vi "Data Logger Main.vi"(0 "Server Data":cluster{"Concat Data":bool, "WebDAV Push":bool}, 1 "In Spec":bool[](array[boolean])=[FALSE, FALSE, FALSE, FALSE, FALSE, FALSE], 2 "Current Step":i32=2, 3 "Step Time Left":dbl=0.21101045608520508, 4 "Pump Data":T4={"Voltages"=[0.015201568603515625, 0.00335693359375, 0.003021240234375, 0.12260055541992188, 0.06085968017578125, 0.052234649658203125], "PumpCurrent"=[0.015201568603515625, 0.00335693359375, 0.003021240234375, 0.12260055541992188, 0.06085968017578125, 0.052234649658203125], "Speed"=[0.0, 0.0, 0.0, 0.0, 0.0, 0.0], "ControllerCurrent"=[0.015201568603515625, 0.00335693359375, 0.003021240234375, 0.12260055541992188, 0.06085968017578125, 0.052234649658203125], "Pressure"=[0.015201568603515625, 0.00335693359375, 0.003021240234375, 0.12260055541992188, 0.06085968017578125, 0.052234649658203125], "Flow"=[0.0, 0.0, 0.0, 0.125, 0.0625, 0.0625], "Elapsed Time (Display)"=[7.1, 7.1, 7.1, 458133.45, 458138.85000000003, 458126.75], "Avg Pressure"=0.0, "Avg Speed"=0.0, "Elapsed Time"=[4074.9003000000002, 4074.9003000000002, 4074.9003000000002, 4074.9003000000002, 4074.9003000000002, 4074.9003000000002]} {"Elapsed Time" format="%<%H:%M:%S>t"; "Elapsed Time (Display)" format="%<%H:%M:%S>t"; "Speed" format="%#_4f"; "ControllerCurrent" format="%#.1g"; "Pressure" format="%#.0f"; "Flow" format="%#.0f"; "PumpCurrent" format="%#.1g"; "Voltages" format="%#.0f"}, 5 "Tank Data":T3 {"PS Actual (V):" format="%.2f"; "Temp1" format="%#_2g"; "Temp2" format="%#_2g"}, 6 "Auxiliary Data":T1={"Diagnostic Reading"=[nan, nan, nan, nan, nan, nan], "Auxiliary Flow"=[nan, nan, nan, nan, nan, nan]}, 7 "Record Time (sec)":dbl, 8 "Data Logger Mode":T9=enum."Main", 9 "Data Log Start":T5={"App Config"={"Location"="", "Profiles Path"=path "", "Current Profile"="", "CA Number"="", "Controller Type:"=enum."Kuhnke", "Stagger Time (ms)"=0, "Tank 1 Fuel"="", "Tank 2 Fuel"="", "Serial Numbers"={"Position 1 SN"="", "Position 2 SN"="", "Poaition 3 SN"="", "Position 4 SN"="", "Position 5 SN"="", "Position 6 SN"=""}, "Pumps Present"={"Pump 1"=FALSE, "Pump 2"=FALSE, "Pump 3"=FALSE, "Pump 4"=FALSE, "Pump 5"=FALSE, "Pump 6"=FALSE}, "VoltCtrlRef"="", "VoltageSelect"=FALSE, "Watlow Present"=FALSE, "Temp 1"=0.0, "Temp 2"=0.0, "V_Run PI?"=FALSE, "Voltage Limits"={"V_Step"=1e-05, "V_CmdMax"=0.0, "V_CmdMin"=0.0}, "Voltage Far PI"={"V_FarSlew"=10.0, "V_FarKp"=0.0, "V_FarKi"=0.0}, "Voltage Mid PI"={"V_MidSlew"=10.0, "V_MidKp"=0.0, "V_MidKi"=0.0}, "Voltage Close PI"={"V_CloseSlew"=10.0, "V_CloseKp"=0.0, "V_CloseKi"=0.0}, "Voltage Scale"={"V_FFm"=10.0, "V_FFb"=0.0}, "Voltage Cutoffs"={"V_MidCutoff"=0.0, "V_CloseCutoff"=0.0}, "Pressure Scale"={"Pres_FFm"=0.0, "Pres_FFb"=0.0}, "Temp Format"=0, "Temp Tolerance"=0.0, "Target Voltage"=0.0, "Target Pressure"=0.0, "Data Log Init"={"Data Path"=path "", "Data Log Rate (S/s)"=0, "AKLH Rate (Hours/S)"=0.0, "Sync Time Offset (min)"=0, "IP Last 3"=0, "WebDAV IP"=""}, "Email Handler IP"="", "ADC Check"=FALSE, "3 Pump Tank"=FALSE, "Freq Flow?"=FALSE, "Profile Temp Control"=FALSE, "Read Controller Diag"=FALSE, "FFT Min Freq."=0, "FFT Max Freq."=0, "Speed by Current"=FALSE, "Watlow is F4T?"=FALSE, "Test Stop Time"=0.0, "Stop Time Enable"=TRUE, "Timers Include Off-Time"=FALSE}, "Profile"=[], "Controller Type"="", "Tank CMDs"={"PS CMD"=0.0, "Press CMD"=0.0, "Temp 1 CMD"=0.0, "Temp 2 CMD"=0.0, "AO2 CMD"=0.0}}, 11 "Data Log Init":T8, 13 "Tank CMDs":T2) -> ()   [LabVIEW 2013]
uses:
  Data Logger Mode.ctl
  Data Log Init.ctl
  Data Log Start.ctl
  Type Defs/App Config.ctl
  Type Defs/Controller Names.ctl
  Controls/Tank CMDs.ctl
  Controls/Pump Data.ctl
  Controls/Tank Data.ctl
  Type Defs/Auxiliary Data.ctl
  <userlib>/_OpenG.lib/array/array.llb/Remove Duplicates from 1D Array (String)__ogtk.vi
  <userlib>/_OpenG.lib/array/array.llb/Filter 1D Array (String)__ogtk.vi
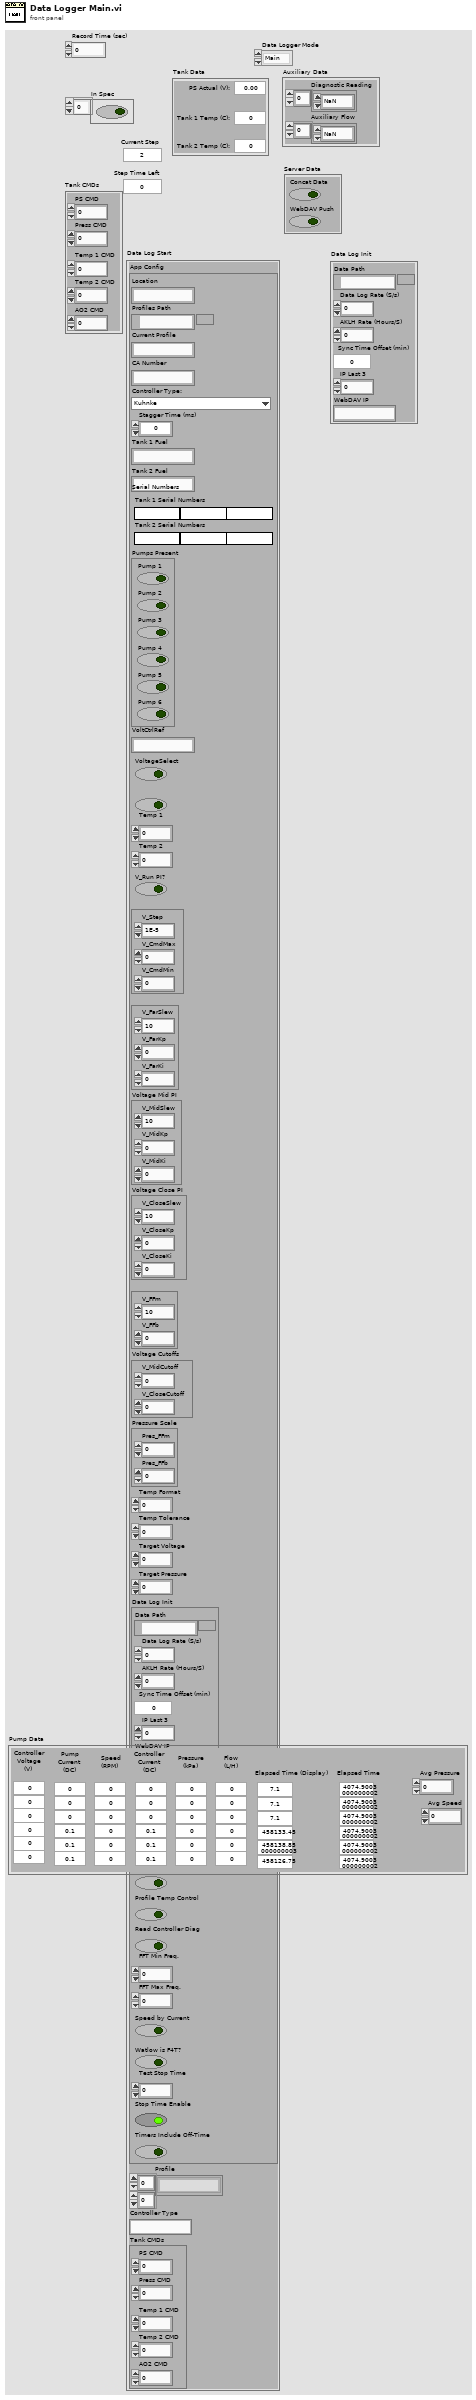
[diagram p1: front panel]
types:
  T1 = typedef "Auxiliary Data.ctl" = cluster{"Diagnostic Reading":dbl[], "Auxiliary Flow":dbl[]}
  T2 = typedef "Tank CMDs.ctl" = cluster{"PS CMD":dbl, "Press CMD":dbl, "Temp 1 CMD":dbl, "Temp 2 CMD":dbl, "AO2 CMD":dbl}
  T3 = typedef "Tank Data.ctl" = cluster{"PS Actual (V):":dbl, "Temp1":dbl, "Temp2":dbl}
  T4 = typedef "Pump Data.ctl" = cluster{"Voltages":dbl[], "PumpCurrent":dbl[], "Speed":dbl[], "ControllerCurrent":dbl[], "Pressure":dbl[], "Flow":dbl[], "Elapsed Time (Display)":dbl[], "Avg Pressure":dbl, "Avg Speed":dbl, "Elapsed Time":dbl[]}
  T5 = typedef "Data Log Start.ctl" = cluster{"App Config":T6, "Profile":string[][], "Controller Type":string, "Tank CMDs":T2}
  T6 = typedef "App Config.ctl" = cluster{"Location":string, "Profiles Path":path, "Current Profile":string, "CA Number":string, "Controller Type:":T7, "Stagger Time (ms)":i32, "Tank 1 Fuel":string, "Tank 2 Fuel":string, "Serial Numbers":cluster{"Position 1 SN":string, "Position 2 SN":string, "Poaition 3 SN":string, "Position 4 SN":string, "Position 5 SN":string, "Position 6 SN":string}, "Pumps Present":cluster{"Pump 1":bool, "Pump 2":bool, "Pump 3":bool, "Pump 4":bool, "Pump 5":bool, "Pump 6":bool}, "VoltCtrlRef":string, "VoltageSelect":bool, "Watlow Present":bool, "Temp 1":dbl, "Temp 2":dbl, "V_Run PI?":bool, "Voltage Limits":cluster{"V_Step":dbl, "V_CmdMax":dbl, "V_CmdMin":dbl}, "Voltage Far PI":cluster{"V_FarSlew":dbl, "V_FarKp":dbl, "V_FarKi":dbl}, "Voltage Mid PI":cluster{"V_MidSlew":dbl, "V_MidKp":dbl, "V_MidKi":dbl}, "Voltage Close PI":cluster{"V_CloseSlew":dbl, "V_CloseKp":dbl, "V_CloseKi":dbl}, "Voltage Scale":cluster{"V_FFm":dbl, "V_FFb":dbl}, "Voltage Cutoffs":cluster{"V_MidCutoff":dbl, "V_CloseCutoff":dbl}, "Pressure Scale":cluster{"Pres_FFm":dbl, "Pres_FFb":dbl}, "Temp Format":i32, "Temp Tolerance":dbl, "Target Voltage":dbl, "Target Pressure":dbl, "Data Log Init":T8, "Email Handler IP":string, "ADC Check":bool, "3 Pump Tank":bool, "Freq Flow?":bool, "Profile Temp Control":bool, "Read Controller Diag":bool, "FFT Min Freq.":i32, "FFT Max Freq.":i32, "Speed by Current":bool, "Watlow is F4T?":bool, "Test Stop Time":dbl, "Stop Time Enable":bool, "Timers Include Off-Time":bool}
  T7 = typedef "Controller Names.ctl" = enum16{"Kuhnke", "Helbako BLDC", "Conti", "Hella BLDC OL PWM", "Hella BLDC Turbine OL PWM", "Hella BLDC Pressure", "Helbako (old)", "TI PWM", "PSA", "Hella Gas", "Hella Diesel", "8 Comm", "10 Comm", "8 Comm Hella", "10 Comm Hella", "8 Comm Omron", "10 Comm Omron", "8 Comm Nissan", "10 Comm Nissan"}
  T8 = typedef "Data Log Init.ctl" = cluster{"Data Path":path, "Data Log Rate (S/s)":u32, "AKLH Rate (Hours/S)":dbl, "Sync Time Offset (min)":i32, "IP Last 3":i32, "WebDAV IP":string}
  T9 = typedef "Data Logger Mode.ctl" = enum16{"Init", "Main", "Start", "Stop"}
  T10 = cluster{"Pump 1":bool, "Pump 2":bool, "Pump 3":bool, "Pump 4":bool, "Pump 5":bool, "Pump 6":bool}
  T11 = cluster{"Data Log Base":path, "AKLH Base":path, "AKLH Today Base":path, "AKLH Sync Base":path, "Data Log Rate (ms)":u32, "AKLH Rate (ms)":u32, "Sync Time (min)":i32, "Profile":string[][], "Target Speeds":string[], "App Config":T6, "AKLH Filenames":string[], "Data Log Dirs":path[], "AKLH Dirs":path[], "AKLH Today Dirs":path[], "AKLH Sync Dirs":path[], "Data Log Hdr Paths":path[], "AKLH Today Hdr Paths":path[], "Log Data":bool, "Data Log Times":u32[], "AKLH Log Times":u32[][], "WebDAV IP":string, "File Check Time (ms)":u32, "File Check Period (ms)":u32, "FC Data Log Times":u32[], "FC AKLH Log Times":u32[][], "Data Log Sizes":i64[], "AKLH Log Sizes":i64[][]}
  T12 = cluster{"Position 1 SN":string, "Position 2 SN":string, "Poaition 3 SN":string, "Position 4 SN":string, "Position 5 SN":string, "Position 6 SN":string}
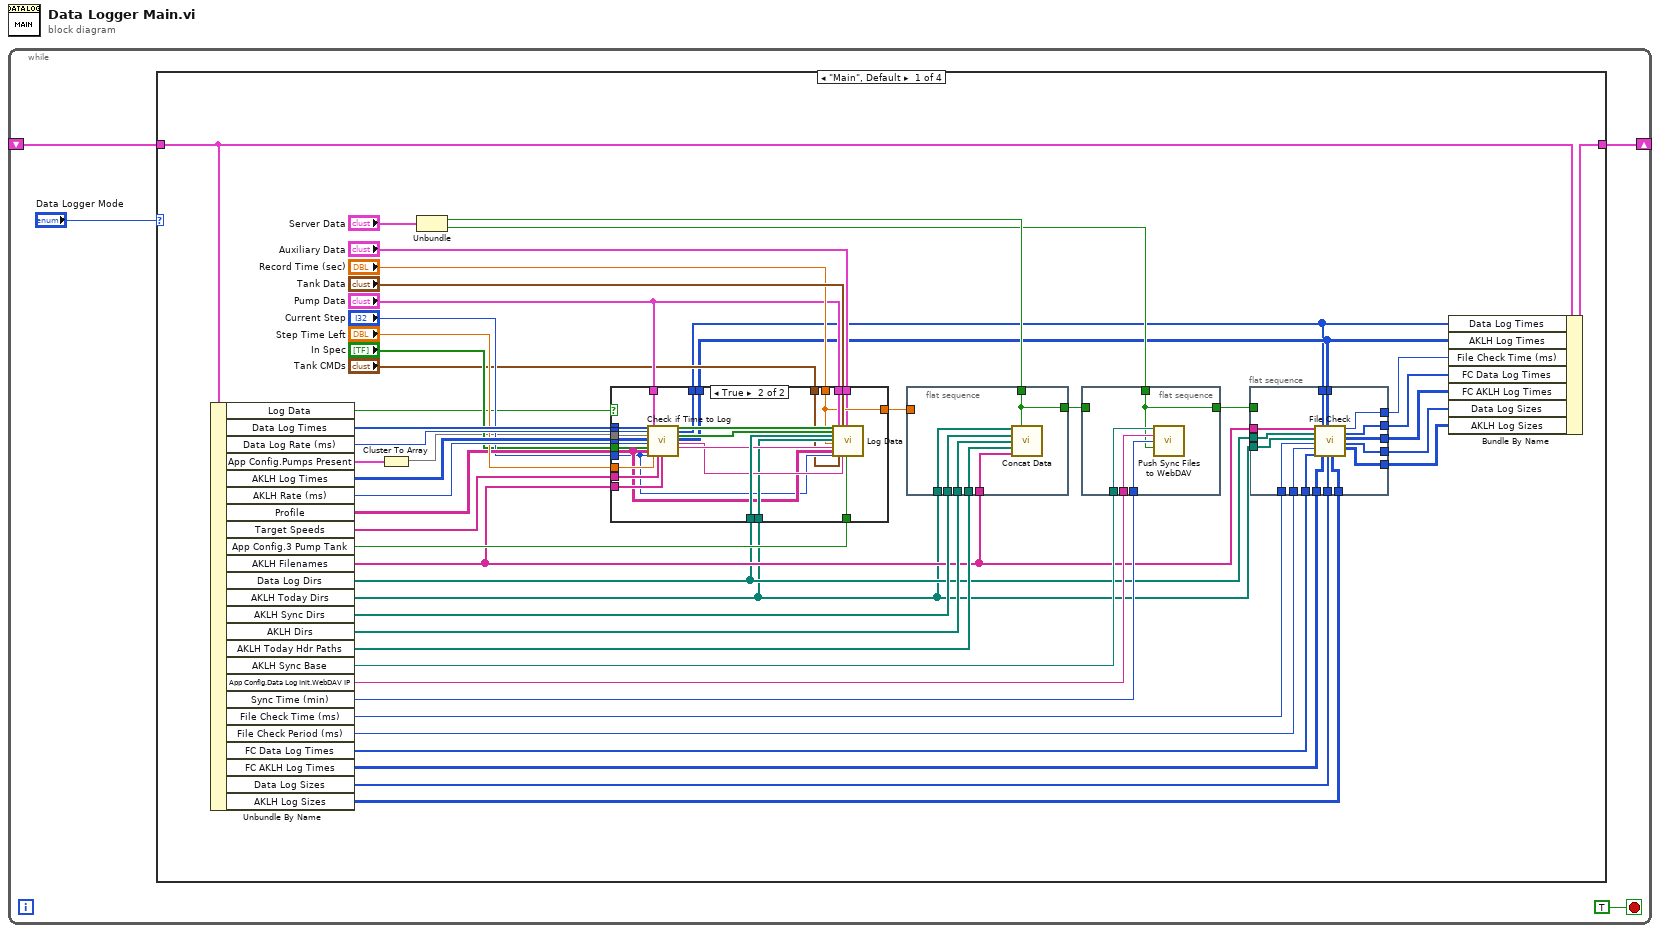
[diagram p0: block diagram]
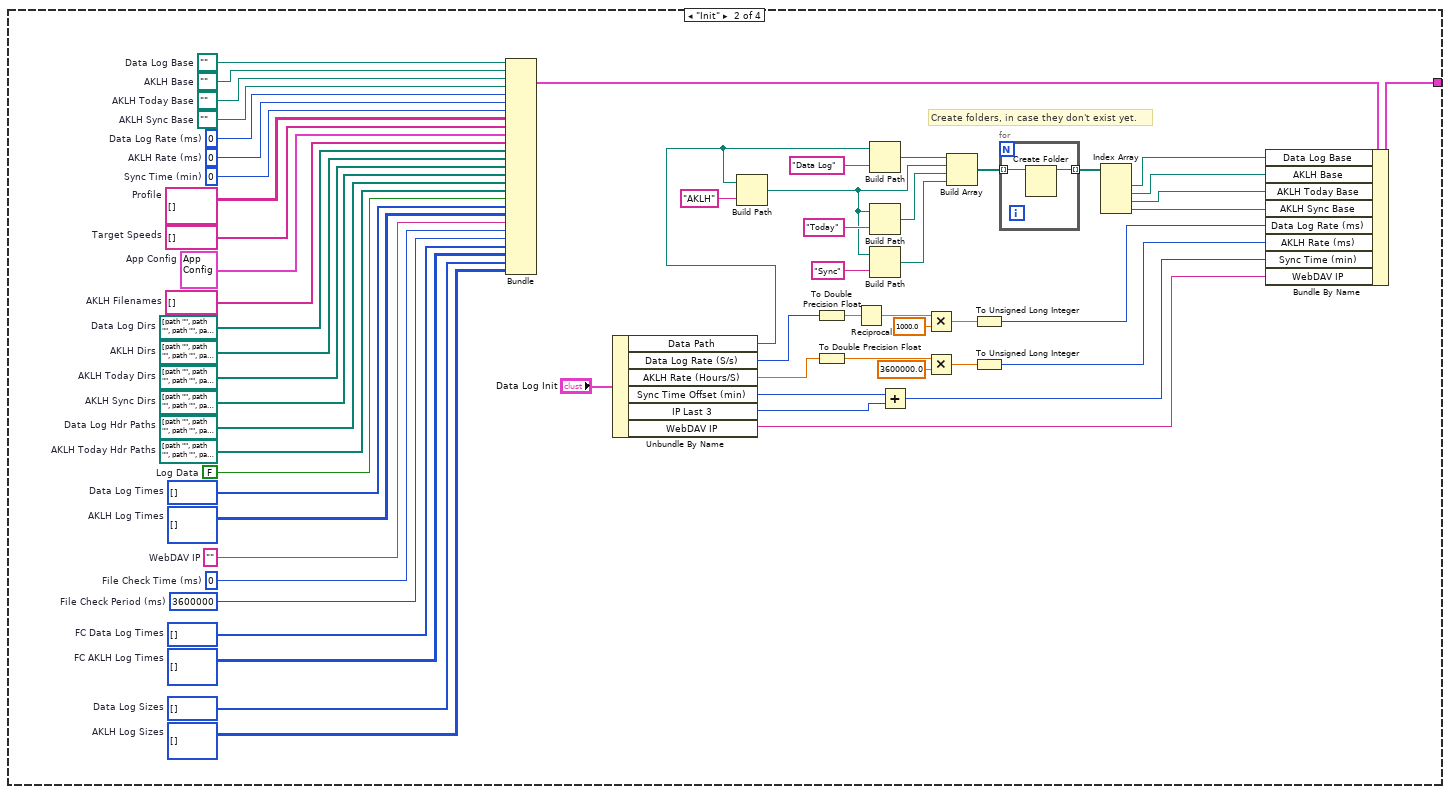
[diagram p3: hidden frame]
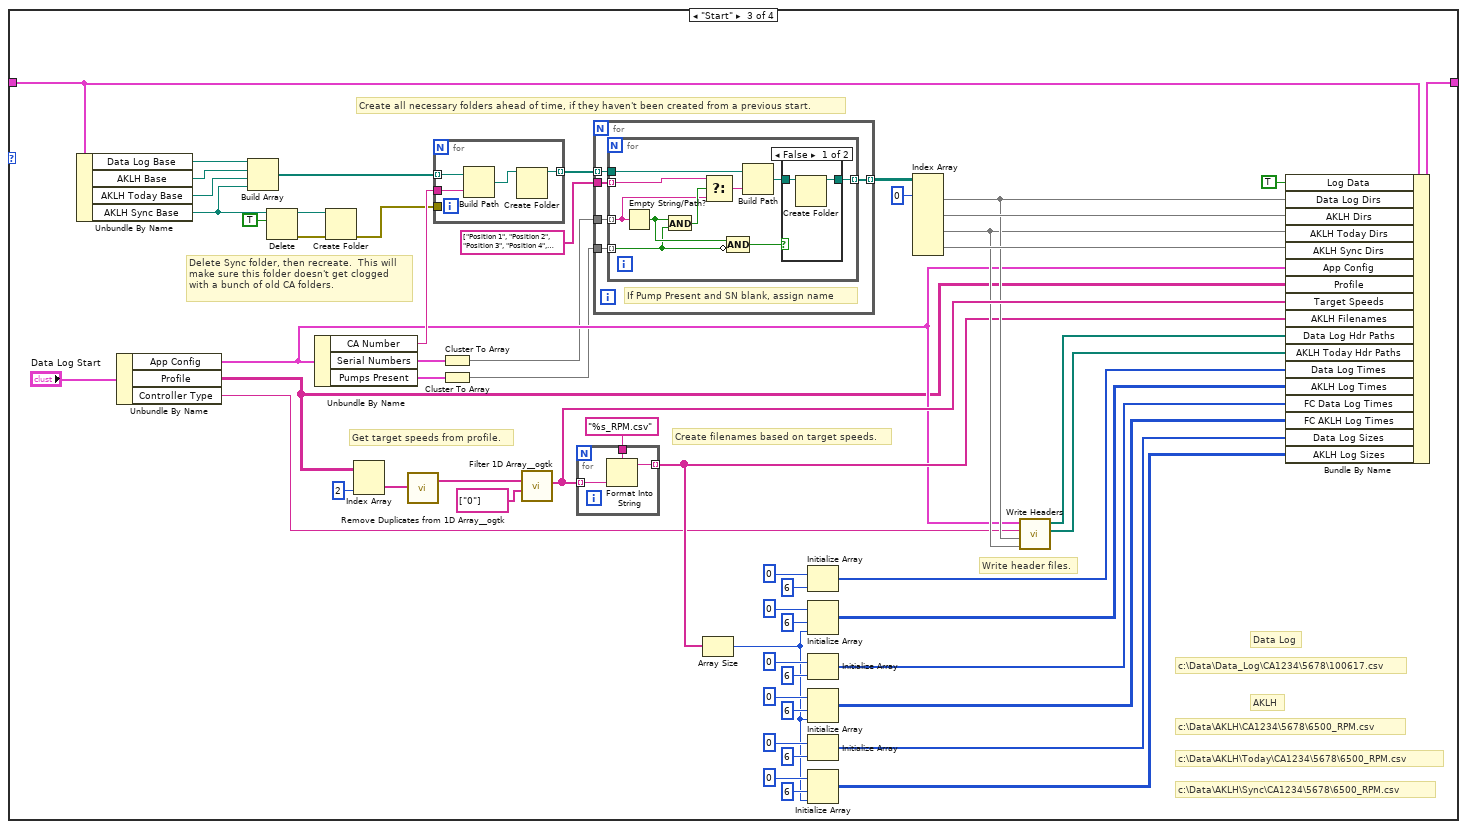
[diagram p4: hidden frame]
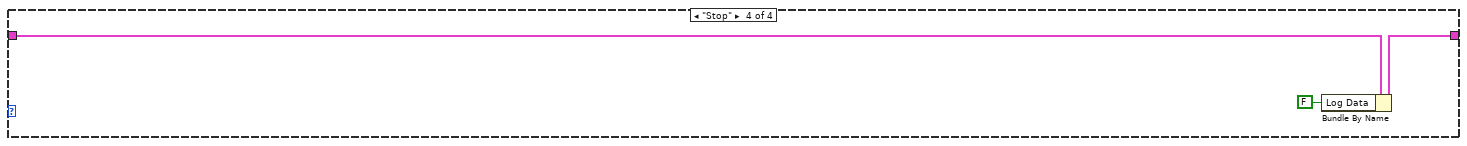
[diagram p6: hidden frame]
diagram:
  n1 = while {
    shift-right: [w2] -> _
    shift-left: _ -> [w1]
    stop <- TRUE stop-if-true
    n2 = case shown="\"Main\", Default" "Data Logger Mode" {
      tunnel: [w51 w160 w212 w253] -> w2
      tunnel: w1 -> [w52 _ w213 w254]
      frame "Main", Default {
        n3 = Unbundle By Name(w52) -> ("Log Data"=w31:bool, "Data Log Times"=w50:u32[], "Data Log Rate (ms)"=w49:u32, "App Config.Pumps Present"=w34:T10, "AKLH Log Times"=w48:u32[][], "AKLH Rate (ms)"=w47:u32, "Profile"=w38:string[][], "Target Speeds"=w45:string[], "App Config.3 Pump Tank"=w28:bool, "AKLH Filenames"=w20:string[], "Data Log Dirs"=w19:path[], "AKLH Today Dirs"=w18:path[], "AKLH Sync Dirs"=w44:path[], "AKLH Dirs"=w43:path[], "AKLH Today Hdr Paths"=w42:path[], "AKLH Sync Base"=w41:path, "App Config.Data Log Init.WebDAV IP"=w40:string, "Sync Time (min)"=w39:i32, "File Check Time (ms)"=w17:u32, "File Check Period (ms)"=w16:u32, "FC Data Log Times"=w15:u32[], "FC AKLH Log Times"=w14:u32[][], "Data Log Sizes"=w13:i64[], "AKLH Log Sizes"=w12:i64[][])
        n4 = Cluster To Array(cluster=w34) -> (array=w33:bool[])
        n5 = Unbundle("Server Data") -> ("Concat Data"=w24:bool, "WebDAV Push"=w23:bool)
        n6 = case shown="True" w31 {
          tunnel: w50 -> [w81 w107]
          tunnel: w49 -> [_ w106]
          tunnel: w48 -> [w80 w105]
          tunnel: w47 -> [_ w104]
          tunnel: "Step Time Left" -> [_ w103]
          tunnel: w45 -> [_ w102]
          tunnel: w19 -> [_ w99]
          tunnel: [w81 w96] -> w10
          tunnel: [w80 w95] -> w11
          tunnel: w18 -> [_ w94]
          tunnel: w20 -> [_ w93]
          tunnel: w38 -> [_ w88]
          tunnel: "Current Step" -> [_ w87]
          tunnel: "Tank Data" -> [_ w92]
          tunnel: "Pump Data" -> [_ w91]
          tunnel: "In Spec" -> [_ w90]
          tunnel: w33 -> [_ w89]
          tunnel: "Record Time (sec)" -> [w79 w86]
          tunnel: [w79 w86] -> w29
          tunnel: w28 -> [_ w85]
          tunnel: "Pump Data" -> [_ w84]
          tunnel: "Tank CMDs" -> [_ w83]
          tunnel: "Auxiliary Data" -> [_ w82]
          frame False {
          }
          frame True {
            n7 = call "Check if Time to Log.vi"("Data Log Times IN"=w107, "Data Log Rate (ms)"=w106, "Pumps Present"=w89, "AKLH Log Times IN"=w105, "AKLH Rate (ms)"=w104, "In Spec"=w90, "Profile"=w88, "Current Step"=w87, "Pump Data"=w84, "Step Time Left"=w103, "Target Speeds"=w102, "AKLH Filenames"=w93) -> ("Log Data"=w101:bool[], "Data Log Times OUT"=w96:u32[], "Log AKLH"=w100:bool[], "AKLH Log Times OUT"=w95:u32[][], "AKLH Filename"=w97:string, "Target Speed"=w98:string)  [unwired: 10 in]
            n8 = call "Log Data.vi"("Log Data"=w101, "Log AKLH"=w100, "Data Log Dirs"=w99, "AKLH Today Dirs"=w94, "Record Time (sec)"=w86, "Target Speed"=w98, "Profile"=w88, "Current Step"=w87, "Pump Data"=w91, "Tank CMDs"=w83, "Tank Data"=w92, "AKLH Filename"=w97, "Auxiliary Data"=w82, "3 Pump Tank"=w85) -> ()  [unwired: 14 in]
          }
        }
        n9 = flat-sequence {
          tunnel: w18 -> [w78]
          tunnel: w44 -> [w77]
          tunnel: w43 -> [w76]
          tunnel: w20 -> [w75]
          tunnel: w42 -> [w74]
          tunnel: w24 -> [w73]
          tunnel: [w73] -> w30
          tunnel: w29 -> [_]
          frame #0 {
            n10 = call "Concat Data.vi"("AKLH Today Dirs"=w78, "Concat Data"=w73, "AKLH Sync Dirs"=w77, "AKLH Dirs"=w76, "AKLH Today Hdr Paths"=w74, "AKLH Filenames"=w75) -> ()  [unwired: 10 in]
          }
        }
        n11 = flat-sequence {
          tunnel: w41 -> [w72]
          tunnel: w40 -> [w71]
          tunnel: w39 -> [w70]
          tunnel: w23 -> [w69]
          tunnel: w30 -> [_]
          tunnel: [w69] -> w21
          frame #0 {
            n12 = call "Push Sync Files to WebDAV.vi"("AKLH Sync Base"=w72, "WebDAV IP"=w71, "Sync Time (min)"=w70, "WebDAV Push"=w69) -> ()  [unwired: 12 in]
          }
        }
        n13 = flat-sequence {
          tunnel: w21 -> [_]
          tunnel: w20 -> [w66]
          tunnel: w19 -> [w65]
          tunnel: w18 -> [w64]
          tunnel: w17 -> [w63]
          tunnel: w16 -> [w62]
          tunnel: w15 -> [w61]
          tunnel: w14 -> [w60]
          tunnel: w13 -> [w58]
          tunnel: w12 -> [w59]
          tunnel: w11 -> [w68]
          tunnel: w10 -> [w67]
          tunnel: [w57] -> w9
          tunnel: [w56] -> w5
          tunnel: [w55] -> w6
          tunnel: [w54] -> w8
          tunnel: [w53] -> w7
          frame #0 {
            n14 = call "File Check.vi"("AKLH Filenames"=w66, "Data Log Dirs"=w65, "AKLH Today Dirs"=w64, "File Check Time (ms) In"=w63, "File Check Period (ms)"=w62, "FC Data Log Times In"=w61, "Data Log Times IN"=w67, "FC AKLH Log Times In"=w60, "AKLH Log Times IN"=w68, "Data Log Sizes In"=w58, "AKLH Log Sizes In"=w59) -> ("File Check Time (ms) Out"=w56:u32, "FC Data Log Times Out"=w55:u32[], "FC AKLH Log Times Out"=w53:u32[][], "Data Log Sizes Out"=w54:i64[], "AKLH Log Sizes Out"=w57:i64[][])  [unwired: 4 in]
          }
        }
        n15 = Bundle By Name(cluster=w52, "Data Log Times"=w10, "AKLH Log Times"=w11, "File Check Time (ms)"=w5, "FC Data Log Times"=w6, "FC AKLH Log Times"=w7, "Data Log Sizes"=w8, "AKLH Log Sizes"=w9) -> (w51:T11)
      }
      frame "Init" {
        w108 = i64[][] []  # AKLH Log Sizes
        w109 = i64[] []  # Data Log Sizes
        w110 = u32[][] []  # FC AKLH Log Times
        w111 = u32[] []  # FC Data Log Times
        w112 = u32 3600000  # File Check Period (ms)
        w113 = u32 0  # File Check Time (ms)
        w130 = ""  # WebDAV IP
        w131 = u32[][] []  # AKLH Log Times
        w132 = u32[] []  # Data Log Times
        w133 = FALSE  # Log Data
        w134 = path[] [path "", path "", path "", path "", path "", path ""]  # AKLH Today Hdr Paths
        w135 = path[] [path "", path "", path "", path "", path "", path ""]  # Data Log Hdr Paths
        w136 = path[] [path "", path "", path "", path "", path "", path ""]  # AKLH Sync Dirs
        w137 = path[] [path "", path "", path "", path "", path "", path ""]  # AKLH Today Dirs
        w138 = path[] [path "", path "", path "", path "", path "", path ""]  # AKLH Dirs
        w139 = path[] [path "", path "", path "", path "", path "", path ""]  # Data Log Dirs
        w140 = string[] []  # AKLH Filenames
        w141 = T6 {"Location"="", "Profiles Path"=path "", "Current Profile"="", "CA Number"="", "Controller Type:"=enum."Kuhnke", "Stagger Time (ms)"=0, "Tank 1 Fuel"="", "Tank 2 Fuel"="", "Serial Numbers"={"Position 1 SN"="", "Position 2 SN"="", "Poaition 3 SN"="", "Position 4 SN"="", "Position 5 SN"="", "Position 6 SN"=""}, "Pumps Present"={"Pump 1"=FALSE, "Pump 2"=FALSE, "Pump 3"=FALSE, "Pump 4"=FALSE, "Pump 5"=FALSE, "Pump 6"=FALSE}, "VoltCtrlRef"="", "VoltageSelect"=FALSE, "Watlow Present"=FALSE, "Temp 1"=0.0, "Temp 2"=0.0, "V_Run PI?"=FALSE, "Voltage Limits"={"V_Step"=0.0, "V_CmdMax"=0.0, "V_CmdMin"=0.0}, "Voltage Far PI"={"V_FarSlew"=0.0, "V_FarKp"=0.0, "V_FarKi"=0.0}, "Voltage Mid PI"={"V_MidSlew"=0.0, "V_MidKp"=0.0, "V_MidKi"=0.0}, "Voltage Close PI"={"V_CloseSlew"=0.0, "V_CloseKp"=0.0, "V_CloseKi"=0.0}, "Voltage Scale"={"V_FFm"=0.0, "V_FFb"=0.0}, "Voltage Cutoffs"={"V_MidCutoff"=0.0, "V_CloseCutoff"=0.0}, "Pressure Scale"={"Pres_FFm"=0.0, "Pres_FFb"=0.0}, "Temp Format"=0, "Temp Tolerance"=0.0, "Target Voltage"=0.0, "Target Pressure"=0.0, "Data Log Init"={"Data Path"=path "", "Data Log Rate (S/s)"=0, "AKLH Rate (Hours/S)"=0.0, "Sync Time Offset (min)"=0, "IP Last 3"=0, "WebDAV IP"=""}, "Email Handler IP"="", "ADC Check"=FALSE, "3 Pump Tank"=FALSE, "Freq Flow?"=FALSE, "Profile Temp Control"=FALSE, "Read Controller Diag"=FALSE, "FFT Min Freq."=0, "FFT Max Freq."=0, "Speed by Current"=FALSE, "Watlow is F4T?"=FALSE, "Test Stop Time"=0.0, "Stop Time Enable"=FALSE, "Timers Include Off-Time"=FALSE}  # App Config
        w143 = string[][] []  # Profile
        w142 = string[] []  # Target Speeds
        w145 = 0  # Sync Time (min)
        w162 = u32 0  # AKLH Rate (ms)
        w163 = u32 0  # Data Log Rate (ms)
        w164 = path ""  # AKLH Sync Base
        w165 = path ""  # AKLH Today Base
        w166 = path ""  # AKLH Base
        w167 = path ""  # Data Log Base
        # "Create folders, in case they don't exist yet."
        n16 = Bundle("Data Log Base"=w167, "AKLH Base"=w166, "AKLH Today Base"=w165, "AKLH Sync Base"=w164, "Data Log Rate (ms)"=w163, "AKLH Rate (ms)"=w162, "Sync Time (min)"=w145, "Profile"=w143, "Target Speeds"=w142, "App Config"=w141, "AKLH Filenames"=w140, "Data Log Dirs"=w139, "AKLH Dirs"=w138, "AKLH Today Dirs"=w137, "AKLH Sync Dirs"=w136, "Data Log Hdr Paths"=w135, "AKLH Today Hdr Paths"=w134, "Log Data"=w133, "Data Log Times"=w132, "AKLH Log Times"=w131, "WebDAV IP"=w130, "File Check Time (ms)"=w113, "File Check Period (ms)"=w112, "FC Data Log Times"=w111, "FC AKLH Log Times"=w110, "Data Log Sizes"=w109, "AKLH Log Sizes"=w108) -> (w161:T11)  [unwired: 1 in]
        n17 = Unbundle By Name("Data Log Init") -> ("Data Path"=w125:path, "Data Log Rate (S/s)"=w121:u32, "AKLH Rate (Hours/S)"=w116:dbl, "Sync Time Offset (min)"=w126:i32, "IP Last 3"=w127:i32, "WebDAV IP"=w128:string)
        n18 = Build Path(base path=w125, name or relative path="AKLH") -> (appended path=w154:path)
        n19 = To Double Precision Float(number=w121) -> (double precision float=w124:dbl)
        n20 = To Double Precision Float(number=w116) -> (double precision float=w115:dbl)
        n21 = Reciprocal(x=w124) -> (1/x=w123:dbl)
        n22 = Build Path(base path=w125, name or relative path="Data Log") -> (appended path=w155:path)
        n23 = Build Path(base path=w154, name or relative path="Today") -> (appended path=w153:path)
        n24 = Build Path(base path=w154, name or relative path="Sync") -> (appended path=w152:path)
        n25 = Add(x=w126, y=w127) -> (x+y=w144:i32)
        n26 = Multiply(x=w123, y=1000.0) -> (x*y=w120:dbl)
        n27 = Multiply(x=w115, y=3600000.0) -> (x*y=w118:dbl)
        n28 = Build Array(w155, w154, w153, w152) -> (w151:path[])
        n29 = To Unsigned Long Integer(number=w120) -> (unsigned 32bit integer=w119:u32)
        n30 = To Unsigned Long Integer(number=w118) -> (unsigned 32bit integer=w114:u32)
        n31 = for {
          tunnel: w151 -> [w169] mode=indexing
          tunnel: [w168] -> w150 mode=indexing
          n32 = Create Folder(path (use dialog)=w169) -> (created path=w168:path)  [unwired: 2 in, 2 out]
        }
        n33 = Index Array(array=w150) -> (element #1=w149:path, element #2=w148:path, element #3=w147:path, element #4=w146:path)  [unwired: 4 in]
        n34 = Bundle By Name(cluster=w161, "Data Log Base"=w149, "AKLH Base"=w148, "AKLH Today Base"=w147, "AKLH Sync Base"=w146, "Data Log Rate (ms)"=w119, "AKLH Rate (ms)"=w114, "Sync Time (min)"=w144, "WebDAV IP"=w128) -> (w160:T11)
      }
      frame "Start" {
        # "Delete Sync folder, then recreate.  This will\nmake sure this folder doesn't get clogged \nwith a bunch of old CA folders."
        # "Write header files."
        # "Create filenames based on target speeds."
        # "Get target speeds from profile."
        # "Create all necessary folders ahead of time, if they haven't been created from a previous start."
        # "c:\\Data\\AKLH\\Sync\\CA1234\\5678\\6500_RPM.csv"
        # "c:\\Data\\AKLH\\Today\\CA1234\\5678\\6500_RPM.csv"
        # "c:\\Data\\AKLH\\CA1234\\5678\\6500_RPM.csv"
        # "AKLH"
        # "Data Log"
        # "c:\\Data\\Data_Log\\CA1234\\5678\\100617.csv"
        n35 = Unbundle By Name(w213) -> ("Data Log Base"=w221:path, "AKLH Base"=w220:path, "AKLH Today Base"=w219:path, "AKLH Sync Base"=w191:path)
        n36 = Unbundle By Name("Data Log Start") -> ("App Config"=w195:T6, "Profile"=w194:string[][], "Controller Type"=w193:string)
        n37 = Build Array(w221, w220, w219, w191) -> (w218:path[])
        n38 = Delete(path (use dialog)=w191, entire hierarchy (F)=TRUE) -> (deleted path=w189:path, error out=w188:errorcluster)  [unwired: 3 in, 1 out]
        n39 = Unbundle By Name(w195) -> ("CA Number"=w217:string, "Serial Numbers"=w186:T12, "Pumps Present"=w224:T10)
        n40 = Create Folder(path (use dialog)=w189, error in=w188) -> (error out=w187:errorcluster)  [unwired: 1 in, 2 out]
        n41 = Index Array(array=w194, index (col)=2 ("disabled index (col)")) -> (element=w225:string[])  [unwired: 1 in]
        n42 = call-poly <userlib>:"Remove Duplicates from 1D Array__ogtk.vi"("Input Array"=w225) -> ("Output Array"=w222:string[])  [unwired: 1 out]
        n43 = for {
          tunnel: w218 -> [w233] mode=indexing
          tunnel: [w231] -> w216 mode=indexing
          tunnel: w217 -> [w230]
          tunnel: w187 -> [_]
          n44 = Build Path(base path=w233, name or relative path=w230) -> (appended path=w232:path)
          n45 = Create Folder(path (use dialog)=w232) -> (created path=w231:path)  [unwired: 2 in, 2 out]
        }
        n46 = Cluster To Array(cluster=w186) -> (array=w185:string[])
        n47 = Cluster To Array(cluster=w224) -> (array=w184:bool[])
        n48 = call-poly <userlib>:"Filter 1D Array__ogtk.vi"("items to filter"=string[] ["0"], "array"=w222) -> ("filtered array"=w209:string[])  [unwired: 4 in, 1 out]
        n49 = for {
          tunnel: w209 -> [w229] mode=indexing
          tunnel: "%s_RPM.csv" ("format string") -> [w228]
          tunnel: [w227] -> w198 mode=indexing
          n50 = Format Into String(format string=w228, w229) -> (resulting string=w227:string)  [unwired: 2 in, 1 out]
        }
        n51 = for {
          tunnel: w216 -> [w237] mode=indexing
          tunnel: w185 -> [w238]
          tunnel: [w236] -> w215 mode=indexing
          tunnel: w184 -> [w235]
          tunnel: string[] ["Position 1", "Position 2", "Position 3", "Position 4", "Position 5", "Position 6"] -> [w234]
          # "If Pump Present and SN blank, assign name"
          n52 = for {
            tunnel: w238 -> [w240] mode=indexing
            tunnel: w237 -> [w248]
            tunnel: [w246] -> w236 mode=indexing
            tunnel: w235 -> [w243] mode=indexing
            tunnel: w234 -> [w241] mode=indexing
            n53 = Empty String/Path?(string/path=w240) -> (empty?=w244:bool)
            n54 = And(x=w244, y=w243) -> (x .and. y?=w242:bool)
            n55 = Select(t=w241, s=w242, f=w240) -> (s? t:f=w239:string)
            n56 = Compound Arithmetic op=AND(w244, invert w243) -> (w245:bool)
            n57 = Build Path(base path=w248, name or relative path=w239) -> (appended path=w247:path)
            n58 = case shown="False" w245 {
              tunnel: w247 -> [w250 w251]
              tunnel: [w249 w251] -> w246
              frame False {
                n59 = Create Folder(path (use dialog)=w250) -> (created path=w249:path)  [unwired: 2 in, 2 out]
              }
              frame True {
              }
            }
          }
        }
        n60 = Array Size(array=w198) -> (size(s)=w174:i32)
        n61 = Initialize Array(u32 0, 6 ("dimension size")) -> (w201:u32[])
        n62 = Initialize Array(u32 0, 6 ("dimension size"), w174) -> (w197:u32[][])
        n63 = Initialize Array(u32 0, 6 ("dimension size")) -> (w173:u32[])
        n64 = Initialize Array(u32 0, 6 ("dimension size"), w174) -> (w172:u32[][])
        n65 = Initialize Array(i64 0, 6 ("dimension size")) -> (w171:i64[])
        n66 = Initialize Array(i64 0, 6 ("dimension size"), w174) -> (w170:i64[][])
        n67 = Index Array(array=w215, index (row) #1=0 ("disabled index (col)")) -> (element #1=w208:path[], element #2=w211:path[], element #3=w207:path[], element #4=w210:path[])  [unwired: 7 in]
        n68 = call "Write Headers.vi"("AKLH Today Dirs"=w207, "Data Log Dirs"=w208, "Controller Type"=w193, "App Config"=w195) -> ("AKLH Today Header Paths"=w205:path[], "Data Log Header Paths"=w206:path[])  [unwired: 6 in]
        n69 = Bundle By Name(cluster=w213, "Log Data"=TRUE, "Data Log Dirs"=w208, "AKLH Dirs"=w211, "AKLH Today Dirs"=w207, "AKLH Sync Dirs"=w210, "App Config"=w195, "Profile"=w194, "Target Speeds"=w209, "AKLH Filenames"=w198, "Data Log Hdr Paths"=w206, "AKLH Today Hdr Paths"=w205, "Data Log Times"=w201, "AKLH Log Times"=w197, "FC Data Log Times"=w173, "FC AKLH Log Times"=w172, "Data Log Sizes"=w171, "AKLH Log Sizes"=w170) -> (w212:T11)
      }
      frame "Stop" {
        n70 = Bundle By Name(cluster=w254, "Log Data"=FALSE) -> (w253:T11)
      }
    }
  }
